vi "Read Status Message.vi"(8 "error in (no error)":errorcluster, 11 "Status Connection Out":T1) -> (0 "error out":errorcluster, 1 "DTACQ Connection Data Out":T1, 2 "New Status Message":bool, 3 "Module Carrier Status":T2)   [LabVIEW 2017, in "Status Monitor Library.lvlib"]
uses:
  Status Monitor Library.lvlib
  Communications/Typedefs/DTACQ Module Carrier Status.ctl
  Communications/Typedefs/DTACQ Status--Enum.ctl
  Communications/Typedefs/DTACQ Connection Data--Cluster.ctl
  Communications/Communications Library.lvlib
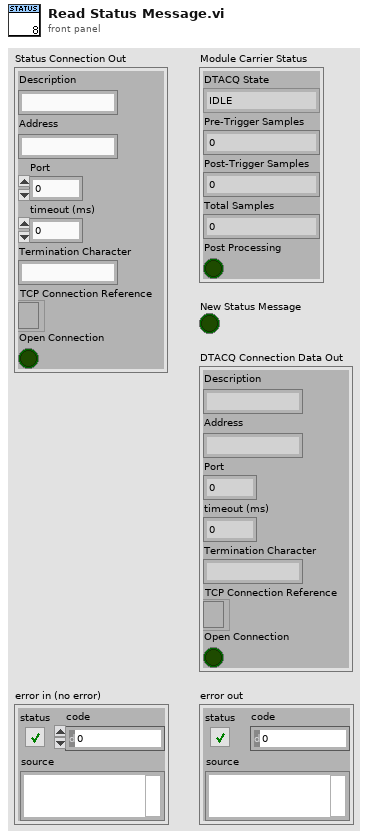
[diagram p1: front panel]
types:
  T1 = typedef "Communications Library.lvlib/DTACQ Connection Data--Cluster.ctl" = cluster{"Description":string, "Address":string, "Port":u16, "timeout (ms)":i32, "Termination Character":string, "TCP Connection Reference":refnum<k5>, "Open Connection":bool}
  T2 = typedef "Communications Library.lvlib/DTACQ Module Carrier Status.ctl" = cluster{"DTACQ State":T3, "Pre-Trigger Samples":i32, "Post-Trigger Samples":i32, "Total Samples":i32, "Post Processing":bool}
  T3 = typedef "Communications Library.lvlib/DTACQ Status--Enum.ctl" = enum16{"IDLE", "ARM", "RUN_PRE-TRIGGER", "RUN_POST-TRIGGER", "POST_PROCESS", "CLEANUP"}
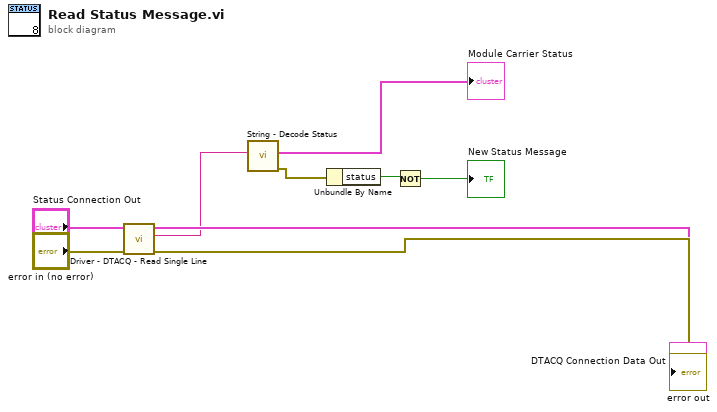
[diagram p0: block diagram]
diagram:
  n1 = call "Driver - DTACQ - Read Single Line.vi"("error in"="error in (no error)", "DTACQ Connection Data In"="Status Connection Out") -> ("error out"=→"error out":errorcluster, "Read String"=w1:string, "DTACQ Connection Data Out"=→"DTACQ Connection Data Out":T1)  [unwired: 6 in, 1 out]
  n2 = call "String - Decode Status.vi"("Status Response String"=w1) -> ("error out"=w3:errorcluster, "Module Carrier Status"=→"Module Carrier Status":T2)  [unwired: 9 in]
  n3 = Unbundle By Name(w3) -> ("status"=w4:bool)
  n4 = Not(x=w4) -> (.not. x?=→"New Status Message":bool)
